vi "PH_Tektronix_7000.set Graph Legend Element.vi"(0 "i ref in":refnum<vi>, 5 "error in (no error)":errorcluster) -> (14 "i ref out":refnum<vi>, 19 "error out":errorcluster)   [LabVIEW 2014, in "PH_Tektronix_7000.lvlib"]
doc: "This sets the Graph Legend Element."
uses:
  PH_Tektronix_7000.lvlib
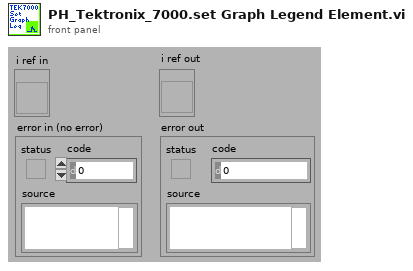
[diagram p1: front panel]
types:
  T1 = typedef "PH_Tektronix_7000.lvlib/PH_Tektronix_7000.i attribute.ctl" = cluster{"VISA Resource Name":refnum<visa-resource-name>, "IDN":cluster{"Instrument Driver":string, "Instrument Firmware":string, "Model":string, "Serial Number":string}, "Selftest":cluster{"Result":i32, "Message":string}, "Trigger Configuration":T2, "Acquisition Configuration":T3, "GUI Refs":T4, "State":T5, "Error Message":string, "Allow Prdc Loop?":bool, "Channel 1":T6, "Channel 2":T6, "Channel 3":T6, "Channel 4":T6, "Data CH 1":waveform(dbl), "Data CH 2":waveform(dbl), "Data CH 3":waveform(dbl), "Data CH 4":waveform(dbl), "Allow config?":bool, "Name Channel 1":string, "Name Channel 2":string, "Name Channel 3":string, "Name Channel 4":string, "Fetch Data before sending to PSDB?":bool, "Constructor passed?":bool, "Data taken at":timestamp, "Plot Colors":u32[], "Default VISA Resource":string}
  T2 = typedef "PH_Tektronix_7000.lvlib/PH_Tektronix_7000.Trigger Config.ctl" = cluster{"Source":u16, "Level [V]":dbl, "Slope":u16, "Coupling":u16, "Trigger Mode":u16}
  T3 = typedef "PH_Tektronix_7000.lvlib/PH_Tektronix_7000.Acquisition Config.ctl" = cluster{"Record Length":u32, "Timebase [s/div]":dbl, "Position [%]":dbl, "Acquisition Type":u16, "Average Waveforms":i32, "Envelope Waveforms":i32, "WfmDB Samples":i32, "Continuous?":bool, "Delay [s]":dbl, "Run?":bool}
  T4 = typedef "PH_Tektronix_7000.lvlib/PH_Tektronix_7000.GUI Refs.ctl" = cluster{"Graph":refnum<vi>, "State":refnum<vi>, "Delete":refnum<vi>, "VISA Resource":refnum<vi>, "Allow Configure":refnum<vi>, "Fetch Data":refnum<vi>, "Fetch before sending Data to PSDB":refnum<vi>, "Name Channel 1":refnum<vi>, "Name Channel 2":refnum<vi>, "Name Channel 3":refnum<vi>, "Name Channel 4":refnum<vi>, "Prdc Intervall [ms]":refnum<vi>, "Data taken":refnum<vi>, "Model":refnum<vi>, "Serial Number":refnum<vi>, "Firmware":refnum<vi>, "Driver":refnum<vi>, "Acquisition":refnum<vi>, "Trigger":refnum<vi>, "Cursor: D Time [s]":refnum<vi>, "Cursor: D Signal [V]":refnum<vi>, "Channel 1":refnum<vi>, "Channel 2":refnum<vi>, "Channel 3":refnum<vi>, "Channel 4":refnum<vi>}
  T5 = typedef "PH_StatusHandler.lvlib/PH_StatusHandler.Status.ctl" = i16
  T6 = typedef "PH_Tektronix_7000.lvlib/PH_Tektronix_7000.Channel Config.ctl" = cluster{"Enable Channel":bool, "Bandwidth":u16, "Input Impedance":u16, "Vertical Coupling":u16, "Probe Attenuation":dbl, "Range [V/div]":dbl, "Position [div]":dbl, "Bandwidth raw":string}
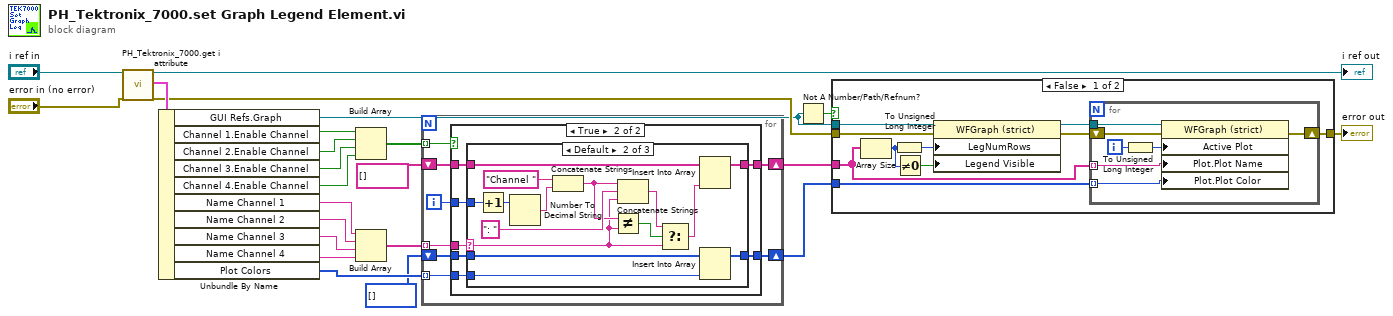
[diagram p0: block diagram]
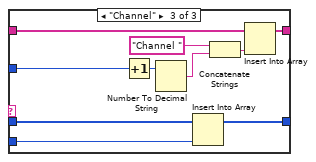
[diagram p4: hidden frame]
diagram:
  n1 = call "PH_Tektronix_7000.get i attribute.vi"("i ref in"="i ref in", "error in (no error)"="error in (no error)") -> ("i ref out"=→"i ref out":refnum<vi>, "i attribute"=w23:T1, "error out"=w22:errorcluster)  [unwired: 15 in]
  n2 = Unbundle By Name(w23) -> ("GUI Refs.Graph"=w4:refnum<vi>, "Channel 1.Enable Channel"=w16:bool, "Channel 2.Enable Channel"=w15:bool, "Channel 3.Enable Channel"=w14:bool, "Channel 4.Enable Channel"=w13:bool, "Name Channel 1"=w12:string, "Name Channel 2"=w11:string, "Name Channel 3"=w10:string, "Name Channel 4"=w9:string, "Plot Colors"=w3:u32[])
  n3 = Build Array(w16, w15, w14, w13) -> (w8:bool[])
  n4 = Build Array(w12, w11, w10, w9) -> (w7:string[])
  n5 = for {
    tunnel: w8 -> [w31] mode=indexing
    tunnel: w7 -> [w30] mode=indexing
    shift-right: [w29] -> w6
    shift-left: string[] [] -> [w28]
    tunnel: w3 -> [w26] mode=indexing
    shift-right: [w25] -> w1
    shift-left: u32[] [] -> [w24]
    i -> [w27]
    n6 = case shown="True" w31 {
      tunnel: w30 -> [_ w37]
      tunnel: [w33 w40] -> w29
      tunnel: w28 -> [w33 w39]
      tunnel: w27 -> [_ w38]
      tunnel: w26 -> [_ w36]
      tunnel: [w32 w35] -> w25
      tunnel: w24 -> [w32 w34]
      frame False {
      }
      frame True {
        n7 = case shown="Default" w37 {
          selector: w37 -> [_ w46 _]
          tunnel: [w42 w57 w67] -> w40
          tunnel: w39 -> [w42 w56 w66]
          tunnel: w38 -> [_ w54 w64]
          tunnel: w36 -> [_ w45 w58]
          tunnel: [w41 w44 w59] -> w35
          tunnel: w34 -> [w41 w43 w60]
          frame "N/A" {
          }
          frame Default {
            n8 = Increment(x=w54) -> (x+1=w53:i32)
            n9 = Number To Decimal String(number=w53) -> (decimal integer string=w52:string)  [unwired: 1 in]
            n10 = Concatenate Strings("Channel " ("string"), w52) -> (w50:string)
            n11 = Not Equal?(x=w50, y=w46) -> (x != y?=w49:bool)
            n12 = Concatenate Strings(w50, ": " ("string"), w46) -> (w48:string)
            n13 = Select(t=w48, s=w49, f=w46) -> (s? t:f=w47:string)
            n14 = Insert Into Array(array=w56, new element=w47) -> (w57:string[])  [unwired: 1 in]
            n15 = Insert Into Array(array=w43, new element=w45) -> (w44:u32[])  [unwired: 1 in]
          }
          frame "Channel" {
            n16 = Increment(x=w64) -> (x+1=w63:i32)
            n17 = Number To Decimal String(number=w63) -> (decimal integer string=w62:string)  [unwired: 1 in]
            n18 = Insert Into Array(array=w60, new element=w58) -> (w59:u32[])  [unwired: 1 in]
            n19 = Concatenate Strings("Channel " ("string"), w62) -> (w61:string)
            n20 = Insert Into Array(array=w66, new element=w61) -> (w67:string[])  [unwired: 1 in]
          }
        }
      }
    }
  }
  n21 = Not A Number/Path/Refnum?(number/path/refnum=w4) -> (NaN/Path/Refnum?=w18:bool)
  n22 = case shown="False" w18 {
    tunnel: w6 -> [w69 _]
    tunnel: w4 -> [w75 _]
    tunnel: w22 -> [w74 w85]
    tunnel: [w73 w85] -> w19
    tunnel: w1 -> [w68 _]
    frame False {
      n23 = Array Size(array=w69) -> (size(s)=w71:i32)
      n24 = To Unsigned Long Integer(number=w71) -> (unsigned 32bit integer=w72:u32)
      n25 = Not Equal To 0?(x=w71) -> (x != 0?=w70:bool)
      n26 = property class="WFGraph (strict)"(reference=w75, error in=w74, "LegNumRows"=w72, "Legend Visible"=w70) -> (reference out=w77:refnum<vi>, error out=w76:errorcluster)
      n27 = for {
        tunnel: w77 -> [w82]
        tunnel: w69 -> [w84] mode=indexing
        shift-right: [w79] -> w73
        shift-left: w76 -> [w80]
        tunnel: w68 -> [w78] mode=indexing
        i -> [w83]
        n28 = To Unsigned Long Integer(number=w83) -> (unsigned 32bit integer=w81:u32)
        n29 = property class="WFGraph (strict)"(reference=w82, error in=w80, "Active Plot"=w81, "Plot.Plot Name"=w84, "Plot.Plot Color"=w78) -> (error out=w79:errorcluster)  [unwired: 1 out]
      }
    }
    frame True {
    }
  }
  "error out" <- w19
